vi "Read Report Path.vi"(11 "Test Report.JUnit in":refnum<class "Test Report.JUnit.lvclass">) -> (2 "Report Path":path, 3 "Test Report.JUnit out":refnum<class "Test Report.JUnit.lvclass">)   [LabVIEW 2009, in "Caraya.lvlib" / "Test Report.JUnit.lvclass"]
uses:
  Test Report.JUnit.lvclass
  Test Report.JUnit.lvclass/Test Report.JUnit.ctl
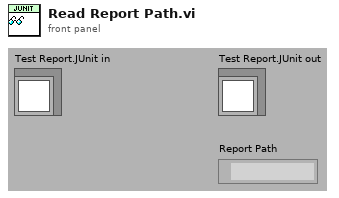
[diagram p1: front panel]
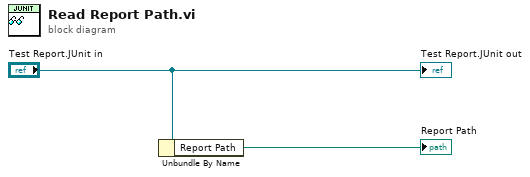
[diagram p0: block diagram]
diagram:
  n1 = Unbundle By Name("Test Report.JUnit in") -> ("Report Path"=→"Report Path":path)
  "Test Report.JUnit out" <- "Test Report.JUnit in"
